vi "Create Shared Variables and Alarms.vi"(8 "error in (no error)":errorcluster, 9 "Alarm Settings":T1(array[cluster]), 10 "Shared Variable Names":string[](array[string])=["PID1-Setpoint", "PID1-Mettler Toledo Scale 1"], 11 "Process Name":string="Flow Module 1") -> (0 "error out":errorcluster, 3 "Shared Variable refnums":refnum<k21>[](array[refnum])=["ni.var.psp://localhost/Flow Module 1/PID1-Setpoint", "ni.var.psp://localhost/Flow Module 1/PID1-Mettler Toledo Scale 1"])   [LabVIEW 2021, in "Dynamic Shared Variables.lvlib"]
uses:
  Dynamic Shared Variables.lvlib
  <vilib>/lvdsc/NI_DSC.lvlib
  <vilib>/lvdsc/variables/internal/Configure Alarming (Shared Variable, Numeric).vi
  <vilib>/lvdsc/variables/internal/Configure Alarming (Shared Variable, Enable Alarming).vi
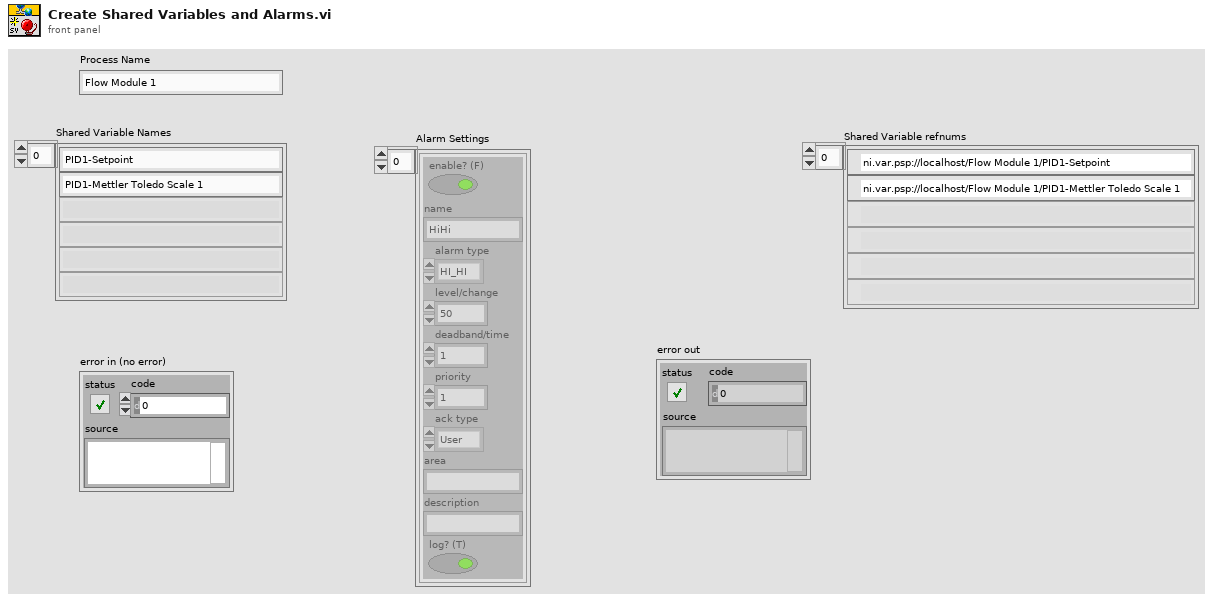
[diagram p1: front panel]
types:
  T1 = cluster{"enable? (F)":bool, "name":string, "alarm type":enum16{"HI_HI", "HI", "LO", "LO_LO"}, "level/change":dbl, "deadband/time":dbl, "priority":u32, "ack type":enum16{"Auto", "User", "None", "Each Occurrence"}, "area":string, "description":string, "log? (T)":bool}[]
  T2 = enum32{"u32BitField", "bool", "double", "string", "int8", "uint8", "int16", "uint16", "int32", "uint32", "int64", "uint64", "single", "double waveform", "int16 waveform", "array of boolean", "array of int8", "array of uint8", "array of int16", "array of uint16", "array of int32", "array of uint32", "array of int64", "array of uint64", "array of single", "array of double", "array of double waveform", "array of int16 waveform", "array of string", "variant", "timestamp", "fixed point", "custom"}
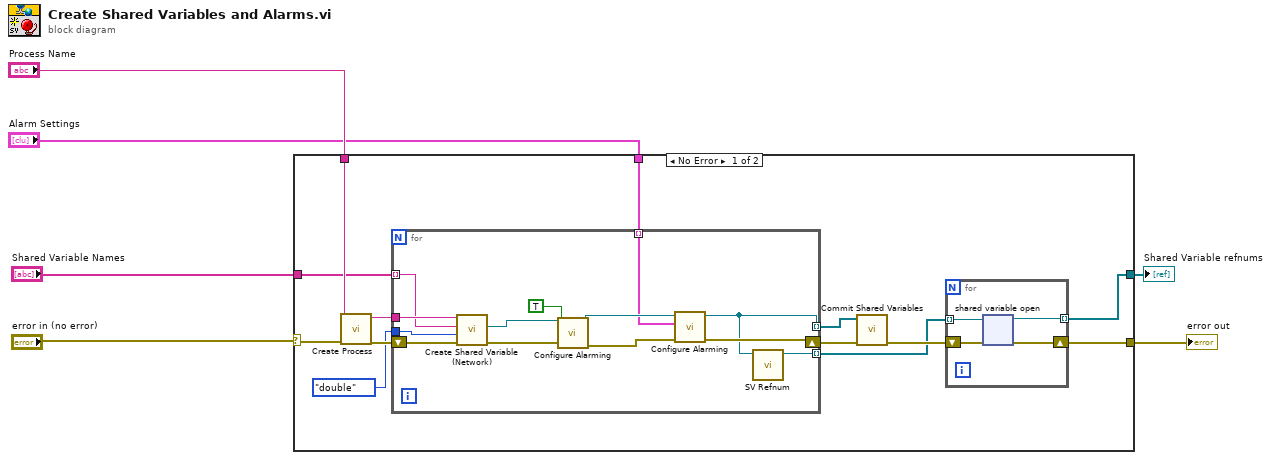
[diagram p0: block diagram]
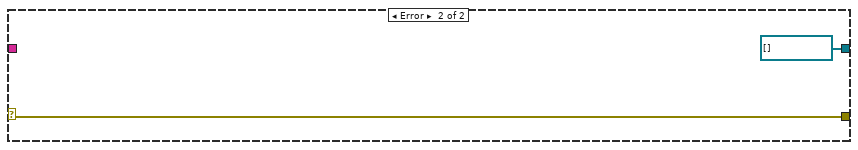
[diagram p2: hidden frame]
diagram:
  n1 = case shown="No Error" "error in (no error)" {
    selector: "error in (no error)" -> [w17 w37]
    tunnel: "Process Name" -> [w19 _]
    tunnel: [w10 w37] -> w4
    tunnel: "Shared Variable Names" -> [w13 _]
    tunnel: [w9 refnum<k21>[] []] -> w2
    tunnel: "Alarm Settings" -> [w7 _]
    frame No Error {
      n2 = call "Create Process.vi"("error in (no error)"=w17, "process name"=w19) -> ("error out"=w18:errorcluster, "dup process name"=w16:string)  [unwired: 8 in]
      n3 = for {
        tunnel: w16 -> [w35]
        shift-right: [w28] -> w14
        shift-left: w18 -> [w36]
        tunnel: [w27] -> w15 mode=indexing
        tunnel: w13 -> [w34] mode=indexing
        tunnel: [w26] -> w11 mode=indexing
        tunnel: T2."double" ("data type") -> [w25]
        tunnel: w7 -> [w24] mode=indexing
        n4 = call "Create Shared Variable (Network).vi"("error in (no error)"=w36, "data type"=w25, "shared variable name"=w34, "process name"=w35) -> ("error out"=w30:errorcluster, "variable reference out"=w31:refnum<k21>)  [unwired: 5 in, 1 out]
        n5 = call-poly <vilib>:"Configure Alarming.vi"("error in (no error)"=w30, "enable? (F)"=TRUE, "variable reference in"=w31) -> ("error out"=w29:errorcluster, "variable reference out"=w32:refnum<k21>)  [unwired: 7 in]
        n6 = call-poly <vilib>:"Configure Alarming.vi"("error in (no error)"=w29, "numeric alarm settings"=w24, "variable reference in"=w32) -> ("error out"=w28:errorcluster, "variable reference out"=w27:refnum<k21>)  [unwired: 7 in]
        n7 = call "SV Refnum.vi"("variable reference in"=w27) -> ("shared variable refnum out"=w26:refnum<k21>)  [unwired: 10 in]
      }
      n8 = call <vilib>:"Commit Shared Variables.vi"("error in (no error)"=w14, "shared variables"=w15) -> ("error out"=w12:errorcluster)  [unwired: 8 in, 1 out]
      n9 = for {
        tunnel: w11 -> [w22] mode=indexing
        tunnel: [w20] -> w9 mode=indexing
        shift-right: [w21] -> w10
        shift-left: w12 -> [w23]
        n10 = shared-variable-open(w22, w23) -> (w20:refnum<k21>, w21:errorcluster)  [unwired: 1 in]
      }
    }
    frame Error {
    }
  }
  "error out" <- w4
  "Shared Variable refnums" <- w2
